vi "Open Reception.vi"(8 "error in (no error)":errorcluster, 11 "TCPIP Communications in":refnum<class "TCPIP Communications.lvclass">) -> (0 "error out":errorcluster, 3 "TCPIP Communications out":refnum<class "TCPIP Communications.lvclass">)   [LabVIEW 2015, in "TCPIP Communications Framework.lvlib" / "TCPIP Communications.lvclass"]
uses:
  TCPIP Communications.lvclass
  TCPIP Communications.lvclass/TCPIP Communications.ctl
  <vilib>/ActorFramework/Actor/Actor.lvclass/Actor.ctl
  <vilib>/ActorFramework/Message Enqueuer/Message Enqueuer.lvclass/Message Enqueuer.ctl
  <vilib>/ActorFramework/Message Enqueuer/Init from Existing Queue.vi
  <vilib>/ActorFramework/Message Enqueuer/Enqueue.vi
  <vilib>/ActorFramework/Message Priority Queue/Priority Enqueue.vi
  <vilib>/ActorFramework/Message Enqueuer/Message Enqueuer.lvclass
  TCPIP Communications Messages/Open Reception Msg/Open Reception Msg.lvclass
  <vilib>/ActorFramework/Actor/Actor.lvclass
  Utilities/Status Messaging.llb/Status Messaging.lvlib
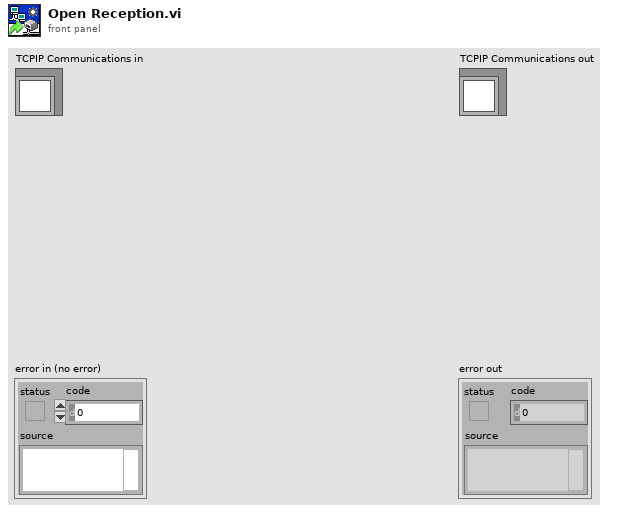
[diagram p1: front panel]
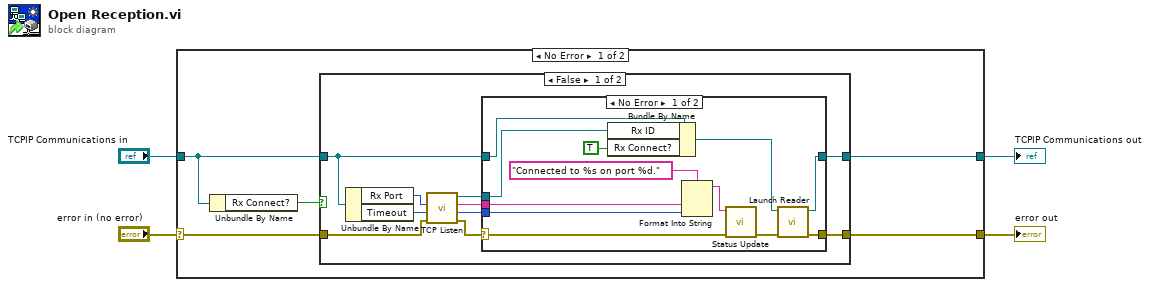
[diagram p0: block diagram]
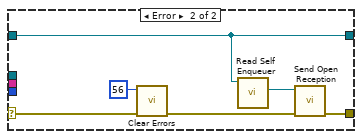
[diagram p2: hidden frame]
diagram:
  n1 = case shown="No Error" "error in (no error)" {
    selector: "error in (no error)" -> [w7 w41]
    tunnel: [w5 w41] -> w3
    tunnel: [w6 w40] -> w1
    tunnel: "TCPIP Communications in" -> [w9 w40]
    frame No Error {
      n2 = Unbundle By Name(w9) -> ("Rx Connect?"=w8:bool)
      n3 = case shown="False" w8 {
        tunnel: w9 -> [w16 w39]
        tunnel: w7 -> [w17 w38]
        tunnel: [w13 w39] -> w6
        tunnel: [w12 w38] -> w5
        frame False {
          n4 = Unbundle By Name(w16) -> ("Rx Port"=w19:u16, "Timeout"=w18:i32)
          n5 = call <vilib>:"TCP Listen.vi"("error in (no error)"=w17, "timeout ms (wait forever: -1)"=w18, "port"=w19) -> ("error out"=w15:errorcluster, "remote port"=w10:u16, "remote address"=w11:string, "connection ID"=w14:refnum<k5>)  [unwired: 4 in, 1 out]
          n6 = case shown="No Error" w15 {
            selector: w15 -> [w25 w37]
            tunnel: w16 -> [w31 w34]
            tunnel: w14 -> [w30 _]
            tunnel: [w27 w34] -> w13
            tunnel: [w26 w32] -> w12
            tunnel: w11 -> [w23 _]
            tunnel: w10 -> [w22 _]
            frame No Error {
              n7 = Bundle By Name(cluster=w31, "Rx ID"=w30, "Rx Connect?"=TRUE ("connected?")) -> (w28:refnum<class "TCPIP Communications.lvclass">)
              n8 = Format Into String(format string="Connected to %s on port %d." ("initial string"), w23, w22) -> (resulting string=w21:string)  [unwired: 2 in, 1 out]
              n9 = call "Status Update.vi"("error in (no error)"=w25, "Status Update"=w21) -> ("error out"=w24:errorcluster)  [unwired: 8 in, 1 out]
              n10 = call "Launch Reader.vi"("error in (no error)"=w24, "TCPIP Communications in"=w28) -> ("error out"=w26:errorcluster, "TCPIP Communications out"=w27:refnum<class "TCPIP Communications.lvclass">)  [unwired: 8 in]
            }
            frame Error {
              n11 = call <vilib>:"Clear Errors.vi"("error in (no error)"=w37, "specific error code to clear (0: all)"=56) -> ("error out"=w33:errorcluster)  [unwired: 4 in, 1 out]
              n12 = call <vilib>:"Read Self Enqueuer.vi"("Actor"=w34) -> ("Self Enqueuer"=w35:refnum<class "Message Enqueuer.lvclass">)  [unwired: 10 in]
              n13 = call "Send Open Reception.vi"("error in (no error)"=w33, "Message Enqueuer"=w35) -> ("error out"=w32:errorcluster)  [unwired: 8 in, 1 out]
            }
          }
        }
        frame True {
        }
      }
    }
    frame Error {
    }
  }
  "error out" <- w3
  "TCPIP Communications out" <- w1
